vi "MB Serial Receive.vi"(7 "Serial Parameters":T1 {"Slave Address" format="%.0x"}, 8 "error in (no error)":errorcluster, 9 "Timeout":u32=10000, 11 "VISA resource name":refnum<visa-resource-name>) -> (0 "error out":errorcluster, 1 "Exception Code":u8 format="%.0x", 2 "Modbus Data Unit":T2={"Function Code"=1, "Data"=[]} {"Function Code" items=["Read Coils"=1, "Read Discrete Inputs"=2, "Read Holding Registers"=3, "Read Input Registers"=4, "Write Single Coil"=5, "Write Single Register"=6, "Read Exception Status"=7, "Write Multiple Coils"=15, "Write Multiple Registers"=16]; "Data" format="%.0x"}, 3 "VISA resource name out":refnum<visa-resource-name>)   [LabVIEW 2017]
uses:
  MB Modbus Data Unit.ctl
panel:
  # "VI Name: MB Serial Receive.vi\nPurpose: Reads a Modbus message.\nReentrant."
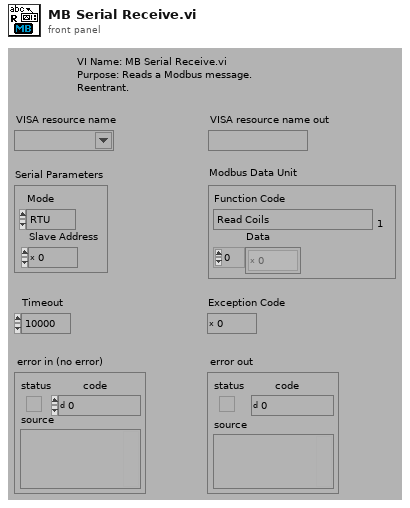
[diagram p1: front panel]
types:
  T1 = cluster{"Mode":enum16{"RTU", "ASCII"}, "Slave Address":u8}
  T2 = typedef "MB Modbus Data Unit.ctl" = cluster{"Function Code":u8, "Data":u8[]}
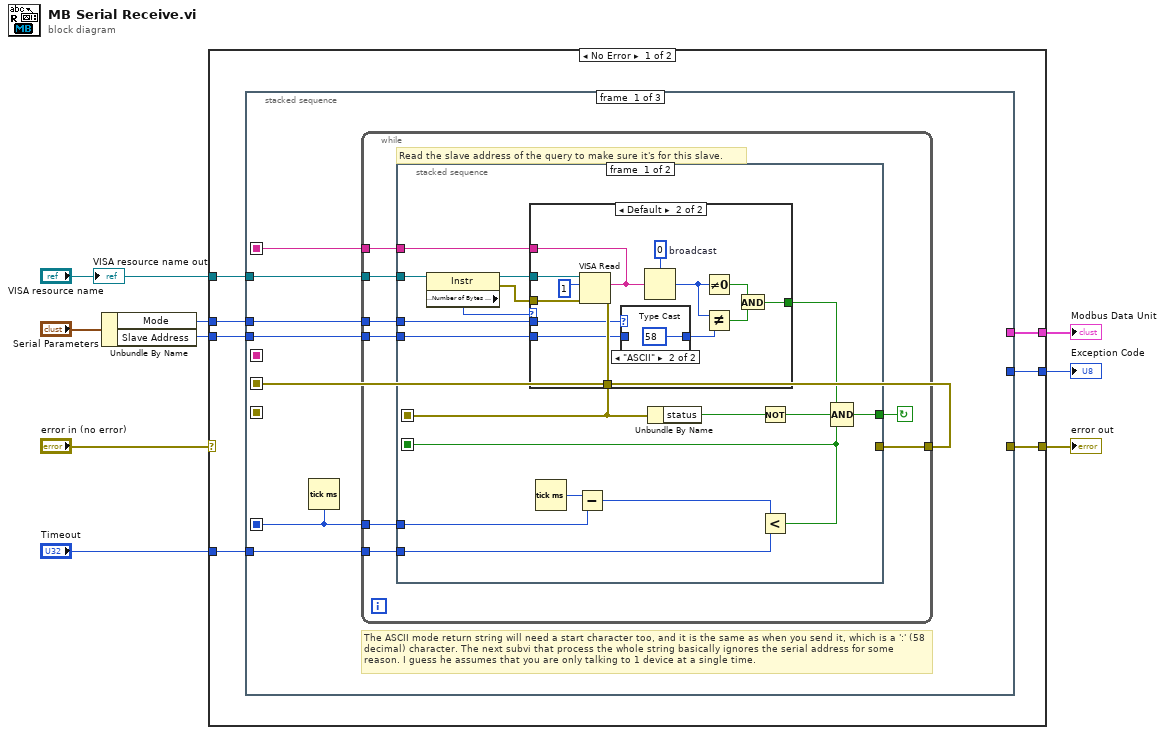
[diagram p0: block diagram]
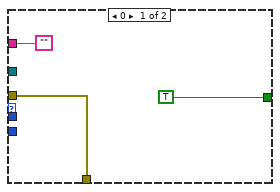
[diagram p2: hidden frame]
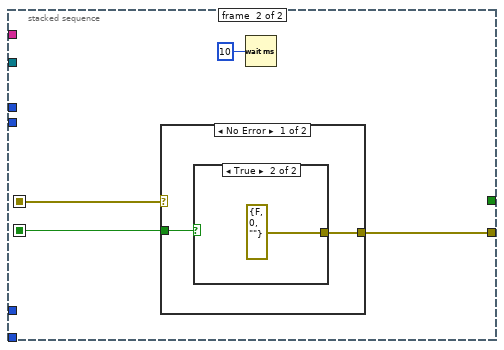
[diagram p4: hidden frame]
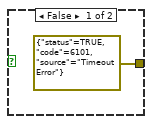
[diagram p5: hidden frame]
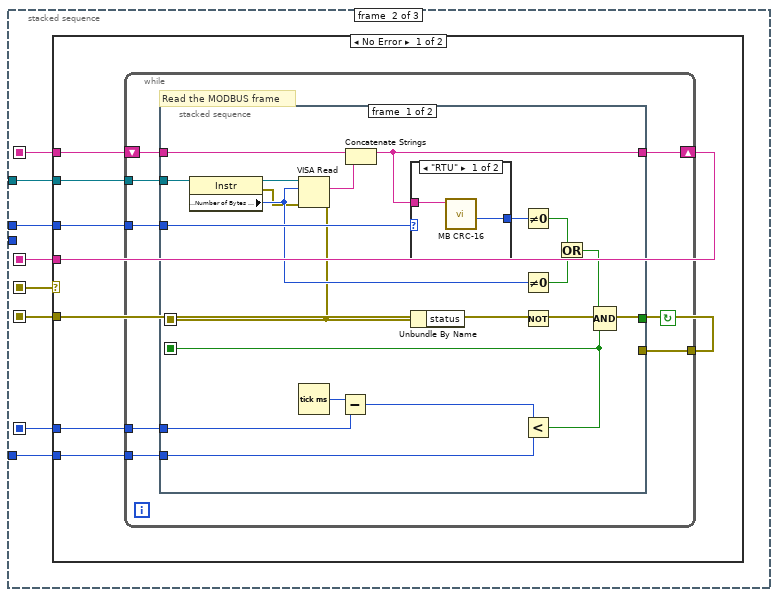
[diagram p7: hidden frame]
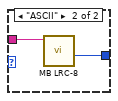
[diagram p8: hidden frame]
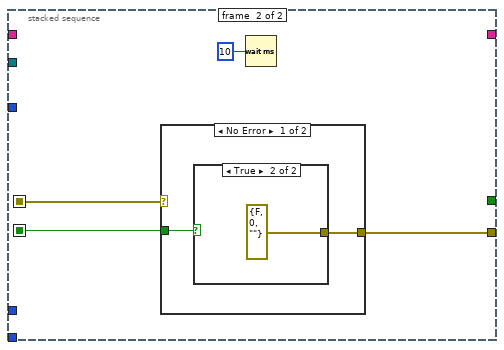
[diagram p9: hidden frame]
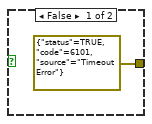
[diagram p10: hidden frame]
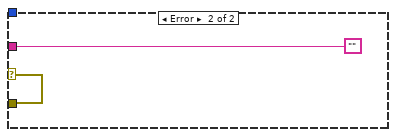
[diagram p12: hidden frame]
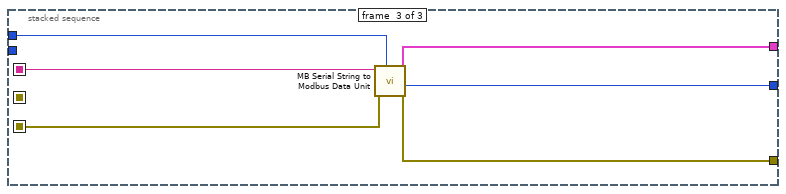
[diagram p13: hidden frame]
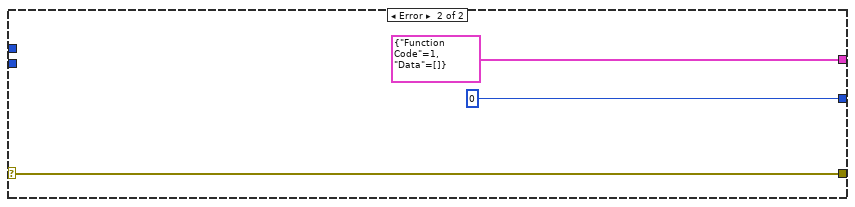
[diagram p14: hidden frame]
diagram:
  n1 = Unbundle By Name("Serial Parameters") -> ("Mode"=w2:enum16{"RTU", "ASCII"}, "Slave Address"=w1:u8)
  n2 = case shown="No Error" "error in (no error)" {
    selector: "error in (no error)" -> [_ w143]
    tunnel: "VISA resource name" -> [w16 _]
    tunnel: w2 -> [w15 _]
    tunnel: [w14 w143] -> w8
    tunnel: [w13 u8 0 ("Exception Code")] -> w6
    tunnel: [w12 T2 {"Function Code"=1, "Data"=[]} ("MODBUS Data Unit")] -> w5
    tunnel: "Timeout" -> [w11 _]
    tunnel: w1 -> [w10 _]
    frame No Error {
      n3 = stacked-sequence {
        seq-local: [_ w81 _] -> [_ _ w138]
        seq-local: [w22 _ _] -> [_ w77 _]
        seq-local: [w20 _ _] -> [_ w79 _]
        seq-local: [_ w78 _] -> [_ _ w135]
        seq-local: [w19 _ _] -> [_ w76 _]
        tunnel: w16 -> [w23 w83 _]
        tunnel: w15 -> [w17 w82 w140]
        tunnel: [_ _ w139] -> w14
        tunnel: [_ _ w137] -> w13
        tunnel: [_ _ w136] -> w12
        tunnel: w11 -> [w21 w80 _]
        tunnel: w10 -> [w18 _ _]
        frame #0 {
          # "The ASCII mode return string will need a start character too, and it is the same as when you send it, which is a ':' (58 decimal) character. The next subvi that process the whole string basically ignores the serial address for some reason. I guess he assumes that you are only talking to 1 device at a single time."
          n4 = Tick Count (ms)() -> (millisecond timer value=w19:u32)
          n5 = while {
            tunnel: w23 -> [w30]
            tunnel: [w29] -> w22
            tunnel: w21 -> [w28]
            tunnel: [w27] -> w20
            tunnel: w19 -> [w26]
            tunnel: w18 -> [w25]
            tunnel: w17 -> [w24]
            stop <- w31 continue-if-true
            # "Read the slave address of the query to make sure it's for this slave."
            n6 = stacked-sequence {
              seq-local: [w41 _] -> [_ w69]
              seq-local: [w40 _] -> [_ w68]
              tunnel: [w48 _] -> w31
              tunnel: w26 -> [w47 _]
              tunnel: w30 -> [w46 _]
              tunnel: [_ w67] -> w29
              tunnel: w28 -> [w39 _]
              tunnel: [w38 _] -> w27
              tunnel: w25 -> [w33 _]
              tunnel: w24 -> [w32 _]
              frame #0 {
                n7 = property class="Instr"(reference=w46) -> (reference out=w45:refnum<visa-resource-name>, error out=w44:errorcluster, "Serial Settings:Number of Bytes at Serial Port"=w37:u32)  [unwired: 1 in]
                n8 = case shown="Default" w37 {
                  tunnel: w45 -> [_ w64]
                  tunnel: w44 -> [w50 w63]
                  tunnel: [w50 w62] -> w41
                  tunnel: ["" w60] -> w38
                  tunnel: [TRUE w55] -> w36
                  tunnel: w33 -> [_ w54]
                  tunnel: w32 -> [_ w52]
                  frame 0 {
                  }
                  frame Default {
                    w59 = u8 0  # broadcast
                    n9 = VISA Read(VISA resource name=w64, byte count=u32 1, error in (no error)=w63) -> (read buffer=w60:string, error out=w62:errorcluster)  [unwired: 2 out]
                    n10 = case shown="\"ASCII\"" w52 {
                      tunnel: w54 -> [w65 _]
                      tunnel: [w65 u8 58 ("Slave Address")] -> w53
                      frame "RTU", Default {
                      }
                      frame "ASCII" {
                      }
                    }
                    n11 = Type Cast(type=w59, x=w60) -> (*(type *) &x=w58:u8)
                    n12 = Not Equal To 0?(x=w58) -> (x != 0?=w57:bool)
                    n13 = Not Equal?(x=w58, y=w53) -> (x != y?=w56:bool)
                    n14 = And(x=w57, y=w56) -> (x .and. y?=w55:bool)
                  }
                }
                n15 = Tick Count (ms)() -> (millisecond timer value=w35:u32)
                n16 = Subtract(x=w35, y=w47) -> (x-y=w34:u32)
                n17 = Unbundle By Name(w41) -> ("status"=w43:bool)
                n18 = Not(x=w43) -> (.not. x?=w42:bool)
                n19 = Less?(x=w34, y=w39) -> (x < y?=w40:bool)
                n20 = Compound Arithmetic op=AND(w36, w42, w40) -> (w48:bool)
              }
              frame #1 {
                n21 = case shown="No Error" w69 {
                  selector: w69 -> [_ w75]
                  tunnel: w68 -> [w72 _]
                  tunnel: [w71 w75] -> w67
                  frame No Error {
                    n22 = case shown="True" w72 {
                      tunnel: [errorcluster {"status"=TRUE, "code"=6101, "source"="Timeout Error"} ("error out") errorcluster {"status"=FALSE, "code"=0, "source"=""} ("error out")] -> w71
                      frame False {
                      }
                      frame True {
                      }
                    }
                  }
                  frame Error {
                  }
                }
                n23 = Wait (ms)(milliseconds to wait=u32 10) -> ()  [unwired: 1 out]
              }
            }
          }
        }
        frame #1 {
          n24 = case shown="No Error" w77 {
            selector: w77 -> [_ w134]
            tunnel: w83 -> [w90 _]
            tunnel: w82 -> [w89 _]
            tunnel: [w88 ""] -> w81
            tunnel: w80 -> [w87 _]
            tunnel: w79 -> [w86 _]
            tunnel: [w85 w134] -> w78
            tunnel: w76 -> [w84 _]
            frame No Error {
              n25 = while {
                tunnel: w89 -> [w97]
                shift-left: w86 -> [w95]
                shift-right: [w92] -> w88
                tunnel: w90 -> [w96]
                tunnel: [w94] -> w85
                tunnel: w87 -> [w93]
                tunnel: w84 -> [w91]
                stop <- w98 continue-if-true
                # "Read the MODBUS frame"
                n26 = stacked-sequence {
                  seq-local: [w102 _] -> [_ w126]
                  seq-local: [w101 _] -> [_ w125]
                  tunnel: [w118 _] -> w98
                  tunnel: w91 -> [w117 _]
                  tunnel: w97 -> [w116 _]
                  tunnel: w96 -> [w111 _]
                  tunnel: w95 -> [w107 _]
                  tunnel: [w105 _] -> w92
                  tunnel: [_ w124] -> w94
                  tunnel: w93 -> [w100 _]
                  frame #0 {
                    n27 = property class="Instr"(reference=w111) -> (reference out=w110:refnum<visa-resource-name>, error out=w108:errorcluster, "Serial Settings:Number of Bytes at Serial Port"=w109:u32)  [unwired: 1 in]
                    n28 = VISA Read(VISA resource name=w110, byte count=w109, error in (no error)=w108) -> (read buffer=w106:string, error out=w102:errorcluster)  [unwired: 2 out]
                    n29 = Tick Count (ms)() -> (millisecond timer value=w119:u32)
                    n30 = Subtract(x=w119, y=w117) -> (x-y=w99:u32)
                    n31 = Concatenate Strings(w107, w106) -> (w105:string)
                    n32 = case shown="\"RTU\"" w116 {
                      tunnel: w105 -> [w121 w123]
                      tunnel: [w120 w122] -> w115
                      frame "RTU" {
                        n33 = call "MB CRC-16.vi"("String"=w121) -> ("CRC-16"=w120:u8)  [unwired: 10 out]
                      }
                      frame "ASCII" {
                        n34 = call "MB LRC-8.vi"("String"=w123) -> ("LRC-8"=w122:u8)  [unwired: 10 out]
                      }
                    }
                    n35 = Unbundle By Name(w102) -> ("status"=w104:bool)
                    n36 = Not Equal To 0?(x=w115) -> (x != 0?=w114:bool)
                    n37 = Not Equal To 0?(x=w109) -> (x != 0?=w112:bool)
                    n38 = Not(x=w104) -> (.not. x?=w103:bool)
                    n39 = Less?(x=w99, y=w100) -> (x < y?=w101:bool)
                    n40 = Or(x=w114, y=w112) -> (x .or. y?=w113:bool)
                    n41 = Compound Arithmetic op=AND(w113, w103, w101) -> (w118:bool)
                  }
                  frame #1 {
                    n42 = case shown="No Error" w126 {
                      selector: w126 -> [_ w132]
                      tunnel: w125 -> [w129 _]
                      tunnel: [w128 w132] -> w124
                      frame No Error {
                        n43 = case shown="True" w129 {
                          tunnel: [errorcluster {"status"=TRUE, "code"=6101, "source"="Timeout Error"} ("error out") errorcluster {"status"=FALSE, "code"=0, "source"=""} ("error out")] -> w128
                          frame False {
                          }
                          frame True {
                          }
                        }
                      }
                      frame Error {
                      }
                    }
                    n44 = Wait (ms)(milliseconds to wait=u32 10) -> ()  [unwired: 1 out]
                  }
                }
              }
            }
            frame Error {
            }
          }
        }
        frame #2 {
          n45 = call "MB Serial String to Modbus Data Unit.vi"("Mode"=w140, "error in (no error)"=w135, "String"=w138) -> ("error out"=w139:errorcluster, "Exception Code"=w137:u8, "Modbus Data Unit"=w136:T2)  [unwired: 1 in, 5 out]
        }
      }
    }
    frame Error {
    }
  }
  "error out" <- w8
  "Exception Code" <- w6
  "Modbus Data Unit" <- w5
  "VISA resource name out" <- "VISA resource name"
